vi "SerialRead.vi"() -> ()   [LabVIEW 2010]
panel:
  out "Position 3":u32
  out "Position 2":u32
  out "Waveform Chart":u16(graph)
  out "Position":u32
  in  "Read":bool
  out "Current String":string
  out "error code":i32
  out "byte count":u32
  out "Read":string
  in  "Quit":bool
  in  "Com Port":i32(ring) items=["Com 0", "Com 1", "Com 2", "Com 3", "Com 4", "Com 5", "Com 6", "COM 7", "COM 8", "COM 9", "COM 10", "COM 11", "COM 12", "com 13", "COM 14"]
  in  "Baud Rate":i32(ring)=2 items=["2400", "4800", "9600", "19200", "38400", "57600", "115200"]
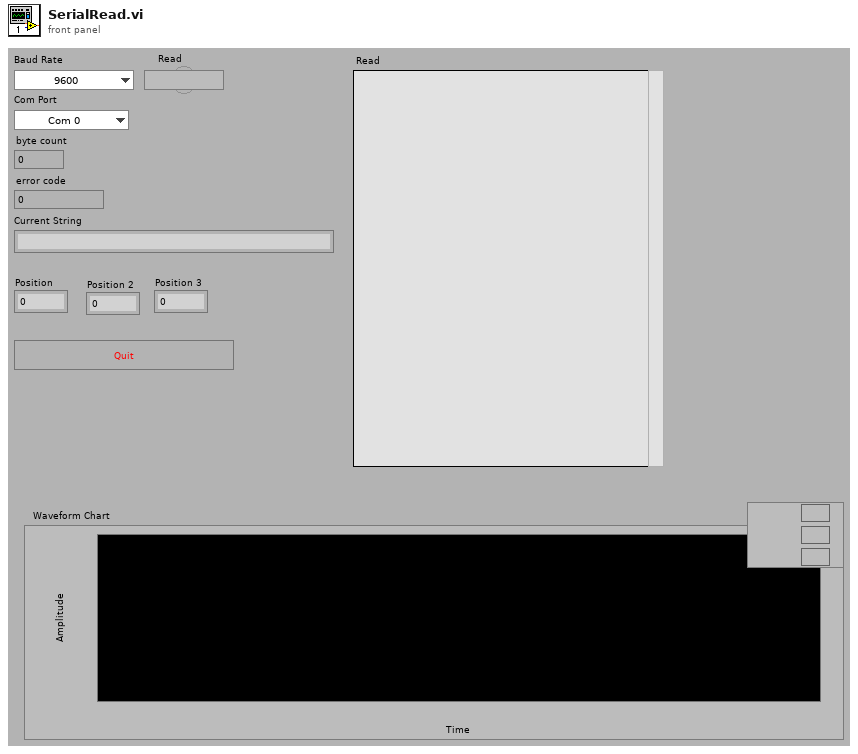
[diagram p1: front panel]
types:
  T1 = enum16{"no parity", "odd parity", "even parity", "mark parity", "space parity"}
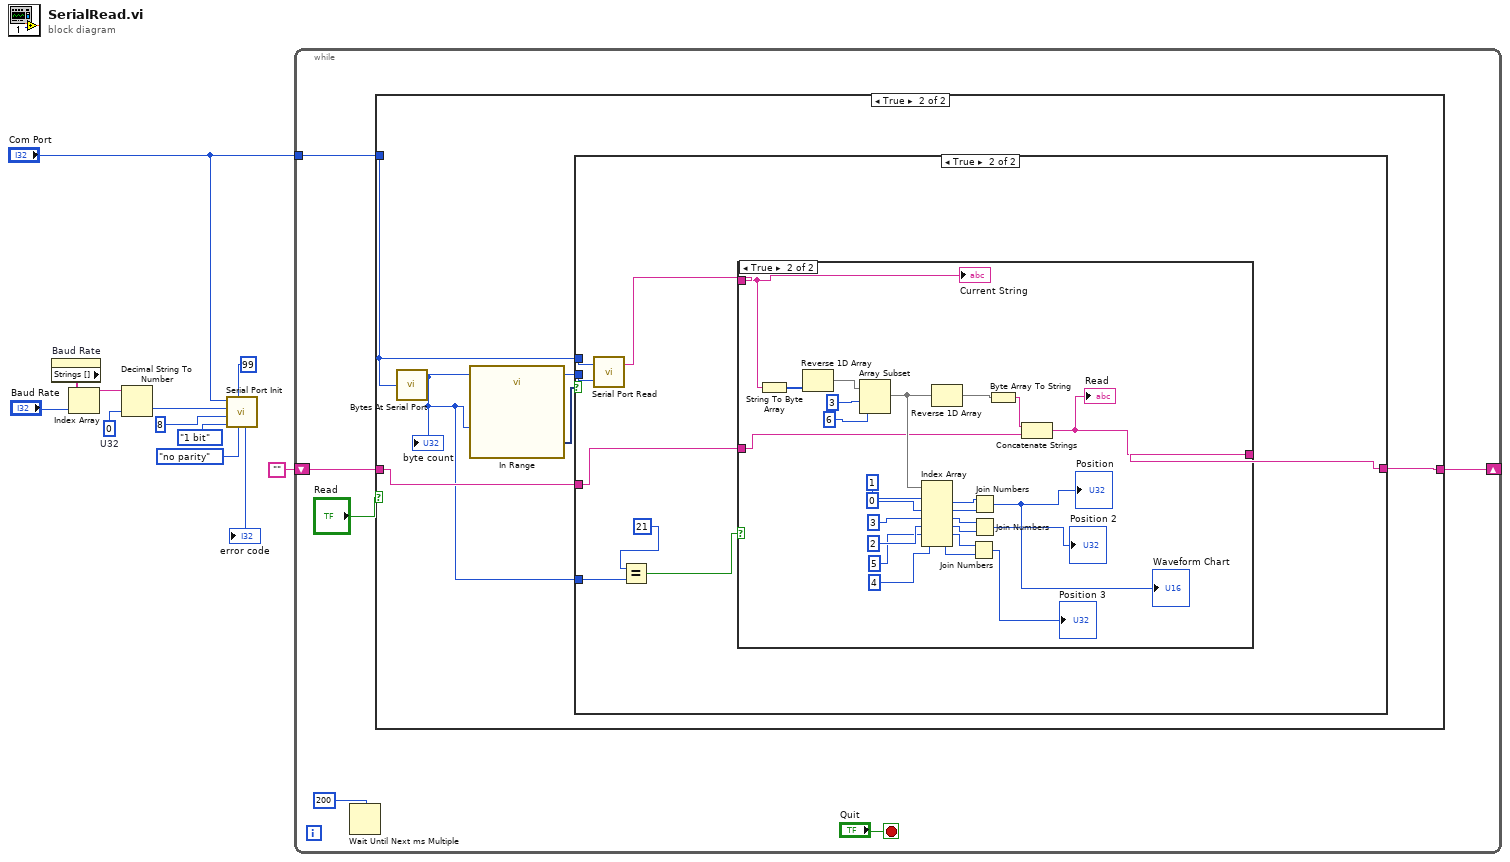
[diagram p0: block diagram]
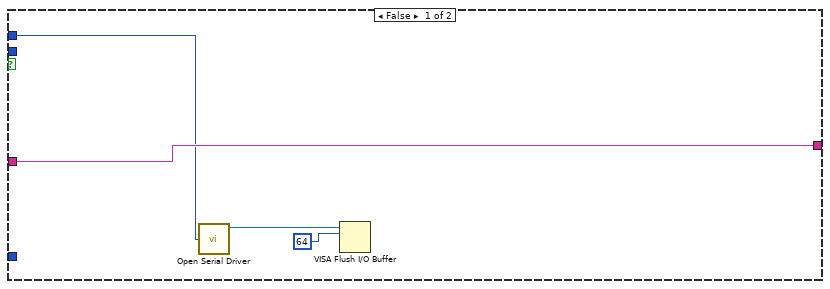
[diagram p3: hidden frame]
diagram:
  w2 = u32 0  # U32
  n1 = property on="Baud Rate" class="Ring (strict)"() -> ("Strings []"=w10:string[])  [unwired: 2 in, 2 out]
  n2 = Index Array(array=w10, index="Baud Rate") -> (element=w9:string)
  n3 = Decimal String To Number(string=w9, default (0L)=w2) -> (number=w1:u32)  [unwired: 2 out]
  n4 = call <vilib>:"Serial Port Init.vi"("parity"=T1."no parity", "buffer size"=u16 99, "stop bits"=enum16{"1 bit", "1.5 bits", "2 bits"}."1 bit", "data bits"=u16 8, "baud rate"=w1, "port number"="Com Port") -> ("error code"=→"error code":i32)  [unwired: 1 in]
  n5 = while {
    shift-left: "" -> [w13]
    shift-right: [w17] -> _
    tunnel: "Com Port" -> [w18]
    stop <- "Quit" stop-if-true
    n6 = Wait Until Next ms Multiple(millisecond multiple=u32 200 ("milliseconds to wait")) -> ()  [unwired: 1 out]
    n7 = case shown="True" "Read" {
      tunnel: w18 -> [_ w24]
      tunnel: w13 -> [w19 w23]
      tunnel: [w19 w20] -> w17
      frame False {
      }
      frame True {
        n8 = call <vilib>:"Bytes At Serial Port.vi"("port number"=w24) -> ("byte count"=w21:u32)  [unwired: 1 out]
        "byte count" <- w21
        n9 = call "In Range"("Operand 1"=w21) -> ("Result"=w22:dynamicdata)  [unwired: 9 in, 1 out]
        n10 = case shown="True" w22 {
          tunnel: w24 -> [w27 w36]
          tunnel: w21 -> [_ w35]
          tunnel: w23 -> [w28 w33]
          tunnel: [w28 w32] -> w20
          tunnel: w21 -> [_ w31]
          frame False {
            n11 = call <vilib>:"Open Serial Driver.vi"("port number"=w27) -> ("input refnum"=w26:refnum<visa-resource-name>)  [unwired: 3 out]
            n12 = VISA Flush I/O Buffer(VISA resource name=w26, mask (16)=64) -> ()  [unwired: 1 in, 2 out]
          }
          frame True {
            n13 = call <vilib>:"Serial Port Read.vi"("requested byte count"=w35, "port number"=w36) -> ("string read"=w34:string)  [unwired: 1 out]
            n14 = Equal?(x=21, y=w31) -> (x = y?=w30:bool)
            n15 = case shown="True" w30 {
              tunnel: w34 -> [_ w50]
              tunnel: w33 -> [w37 w49]
              tunnel: [w37 w48] -> w32
              frame False {
              }
              frame True {
                n16 = String To Byte Array(string=w50) -> (unsigned byte array=w57:u8[])
                n17 = Reverse 1D Array(array=w57) -> (reversed array=w58:u8[])
                n18 = Array Subset(array=w58, index=3, length=6) -> (w59:u8[])
                n19 = Index Array(array=w59, index #1=1, index #2=0, index #3=3, index #4=2, index #5=5, index #6=4) -> (element #1=w56:u8, element #2=w55:u8, element #3=w45:u8, element #4=w44:u8, element #5=w43:u8, element #6=w42:u8)
                n20 = Reverse 1D Array(array=w59) -> (reversed array=w60:u8[])
                n21 = Join Numbers(hi=w43, lo=w42) -> ((hi.lo)=→"Position 3":u16)
                n22 = Join Numbers(hi=w56, lo=w55) -> ((hi.lo)=→"Position" →"Waveform Chart":u16)
                n23 = Join Numbers(hi=w45, lo=w44) -> ((hi.lo)=→"Position 2":u16)
                n24 = Byte Array To String(unsigned byte array=w60) -> (string=w61:string)
                n25 = Concatenate Strings(w61, w49) -> (w48:string)
                "Read" <- w48
                "Current String" <- w50
              }
            }
          }
        }
      }
    }
  }
